vi "Sub Super Duper_2014 05 29_JWa.vi"(0 "VISA resource name":refnum<visa-resource-name>="GPIB0::17::INSTR", 1 "Sample Properties:":T9 {"Date Created" format="%<%Y/%m/%d>T"}, 2 "Gated SMU4 is...":bool, 3 "TRF Cluster":T10={"Step 4"=-38.0, "# of Loops"=1.0, "Transfer 2"=FALSE, "Start 4"=-2.0, "Total Points 2"=2, "Start 3"=40.0, "Stop 2"=-40.0, "Step 3"=-1.0, "Loop Step"=0.0, "Integration Time 3"=0, "Loop Wait"=0.0, "First Step"=0.0} {"Loop Wait" format="%<%H:%M:%S>t"; "Integration Time 3" scale=0.0..2.0; "Step 3" format="%.2f"; "Stop 2" format="%.2f"; "Start 3" format="%.2f"; "Start 4" format="%.2f"; "Step 4" format="%.2f"}, 4 "TSP Cluster":T11={"Transport"=FALSE, "Start 2"=0.0, "Stop 3"=-60.0, "Step 2"=-1.0, "Start"=0.0, "Step"=-10.0, "Total Points"=7, "Integration Time"=0} {"Integration Time" scale=0.0..2.0; "Step" format="%.2f"; "Start" format="%.2f"; "Step 2" format="%.2f"; "Stop 3" format="%.2f"; "Start 2" format="%.2f"}, 5 "Compliance Cluster":T6={"Var1 sweep settings"={"sweep spacing (linear: 0)"=0, "sweep mode"=FALSE, "compliance (V)"=100.0, "compliance (A)"=0.001}, "Var1 sweep settings 2"={"sweep spacing (linear: 0)"=0, "sweep mode"=FALSE, "compliance (V)"=100.0, "compliance (A)"=0.001}, "Var2 step settings 2"={"compliance (A)"=0.001, "compliance (V)"=100.0}, "Var2 step settings"={"compliance (A)"=0.001, "compliance (V)"=100.0}} {"Var2 step settings"."compliance (V)" format="%.2f"; "Var2 step settings"."compliance (A)" format="%^.2e"; "Var2 step settings 2"."compliance (V)" format="%.2f"; "Var2 step settings 2"."compliance (A)" format="%^.2e"; "Var1 sweep settings 2"."compliance (A)" format="%^.2e"; "Var1 sweep settings 2"."compliance (V)" format="%.2f"; "Var1 sweep settings 2"."sweep spacing (linear: 0)" items=["linear", "log 10", "log 25", "log 50"]; "Var1 sweep settings"."compliance (A)" format="%^.2e"; "Var1 sweep settings"."compliance (V)" format="%.2f"; "Var1 sweep settings"."sweep spacing (linear: 0)" items=["linear", "log 10", "log 25", "log 50"]}, 6 "Light Bathe Cluster":T2={"TG to BG:  "=FALSE, "TG to BG Durration"=120.0, "TRF to TSP:   "=FALSE, "TRF to TSP Duration"=120.0, "Post Measure: "=FALSE, "TG to BG (TSP):"=FALSE, "TG to BG Durration 3"=120.0} {"TG to BG Durration 3" format="%<%H:%M:%S>t"; "TRF to TSP Duration" format="%<%H:%M:%S>t"; "TG to BG Durration" format="%<%H:%M:%S>t"}, 7 "error in":errorcluster, 8 "Saved Folder:":path=path "C:/1DATA/2011", 9 "Wait Cluster":T5 {"Wait Time (s)" format="%.1g"; "Wait Countdown" format="%<%H:%M:%S%1u>t"}, 11 "TG Dielectric Prop":T1, 13 "Stop \nCountdown":bool, 15 "Loop Count":dbl, 16 "Gate Current Cluster":T3={"Gate Current (TSP)"={"Y2 axis on/off"=FALSE, "MINIMUM"=0.0, "MAXIMUM"=1.0, "Variable name"="Ig", "LIN or LOG axis"="LIN"}, "Gate Current (TRF)"={"Y2 axis on/off"=FALSE, "MINIMUM"=0.0, "MAXIMUM"=1.0, "Variable name"="Ig", "LIN or LOG axis"="LIN"}} {"Gate Current (TSP)"."MAXIMUM" format="%.9f"; "Gate Current (TSP)"."MINIMUM" format="%.9f"; "Gate Current (TRF)"."MAXIMUM" format="%.9f"; "Gate Current (TRF)"."MINIMUM" format="%.9f"}, 17 "Dielectric Constant (BG)":dbl) -> (12 "Status Indicator":bool, 14 "Vt Cluster":T4 {"Id Max" format="%.3g"; "Vt Max" format="%.3g"; "Vt Min" format="%.3g"; "Vt Ratio" format="%.3g"}, 20 "VISA resource name out":refnum<visa-resource-name>, 21 "TRF Path":path, 23 "TSP Path":path, 24 "Graph Cluster":T7, 25 "Char Cluster":T8 {"Mobility-Lin" format="%#_4e"; "On/Off" format="%#_4e"; "Mobility-Sat" format="%#_4e"}, 27 "error out":errorcluster)   [LabVIEW 2012]
uses:
  <vilib>/Platform/TimedLoop/XDataNode/wakeup.ctl
  <vilib>/Platform/TimedLoop/XDataNode/XDNodeRunTimeDep.lvlib
  <vilib>/Platform/TimedLoop/XDataNode/nitl_modes.ctl
  <vilib>/Platform/TimedLoop/XDataNode/timing_clust.ctl
  <vilib>/Platform/TimedLoop/XDataNode/XDataNode.xnode
panel:
  in  "Ambient Temp (Y/N)":bool=TRUE
  out "LKG Path":path
  # "Vg Sweep"
  # "Vd Step"
  # "Loops and Integration Time"
  # "Device Characteristics"
  # "Light Bath is..."
  # "Duration (hh:mm:ss)"
  # "Sample Properties:"
  # "%"
  # "nm"
  # "Device Properties:"
  # "um"
  # "um"
  # "Vg Step"
  # "Vd Step"
  # "Integration Time"
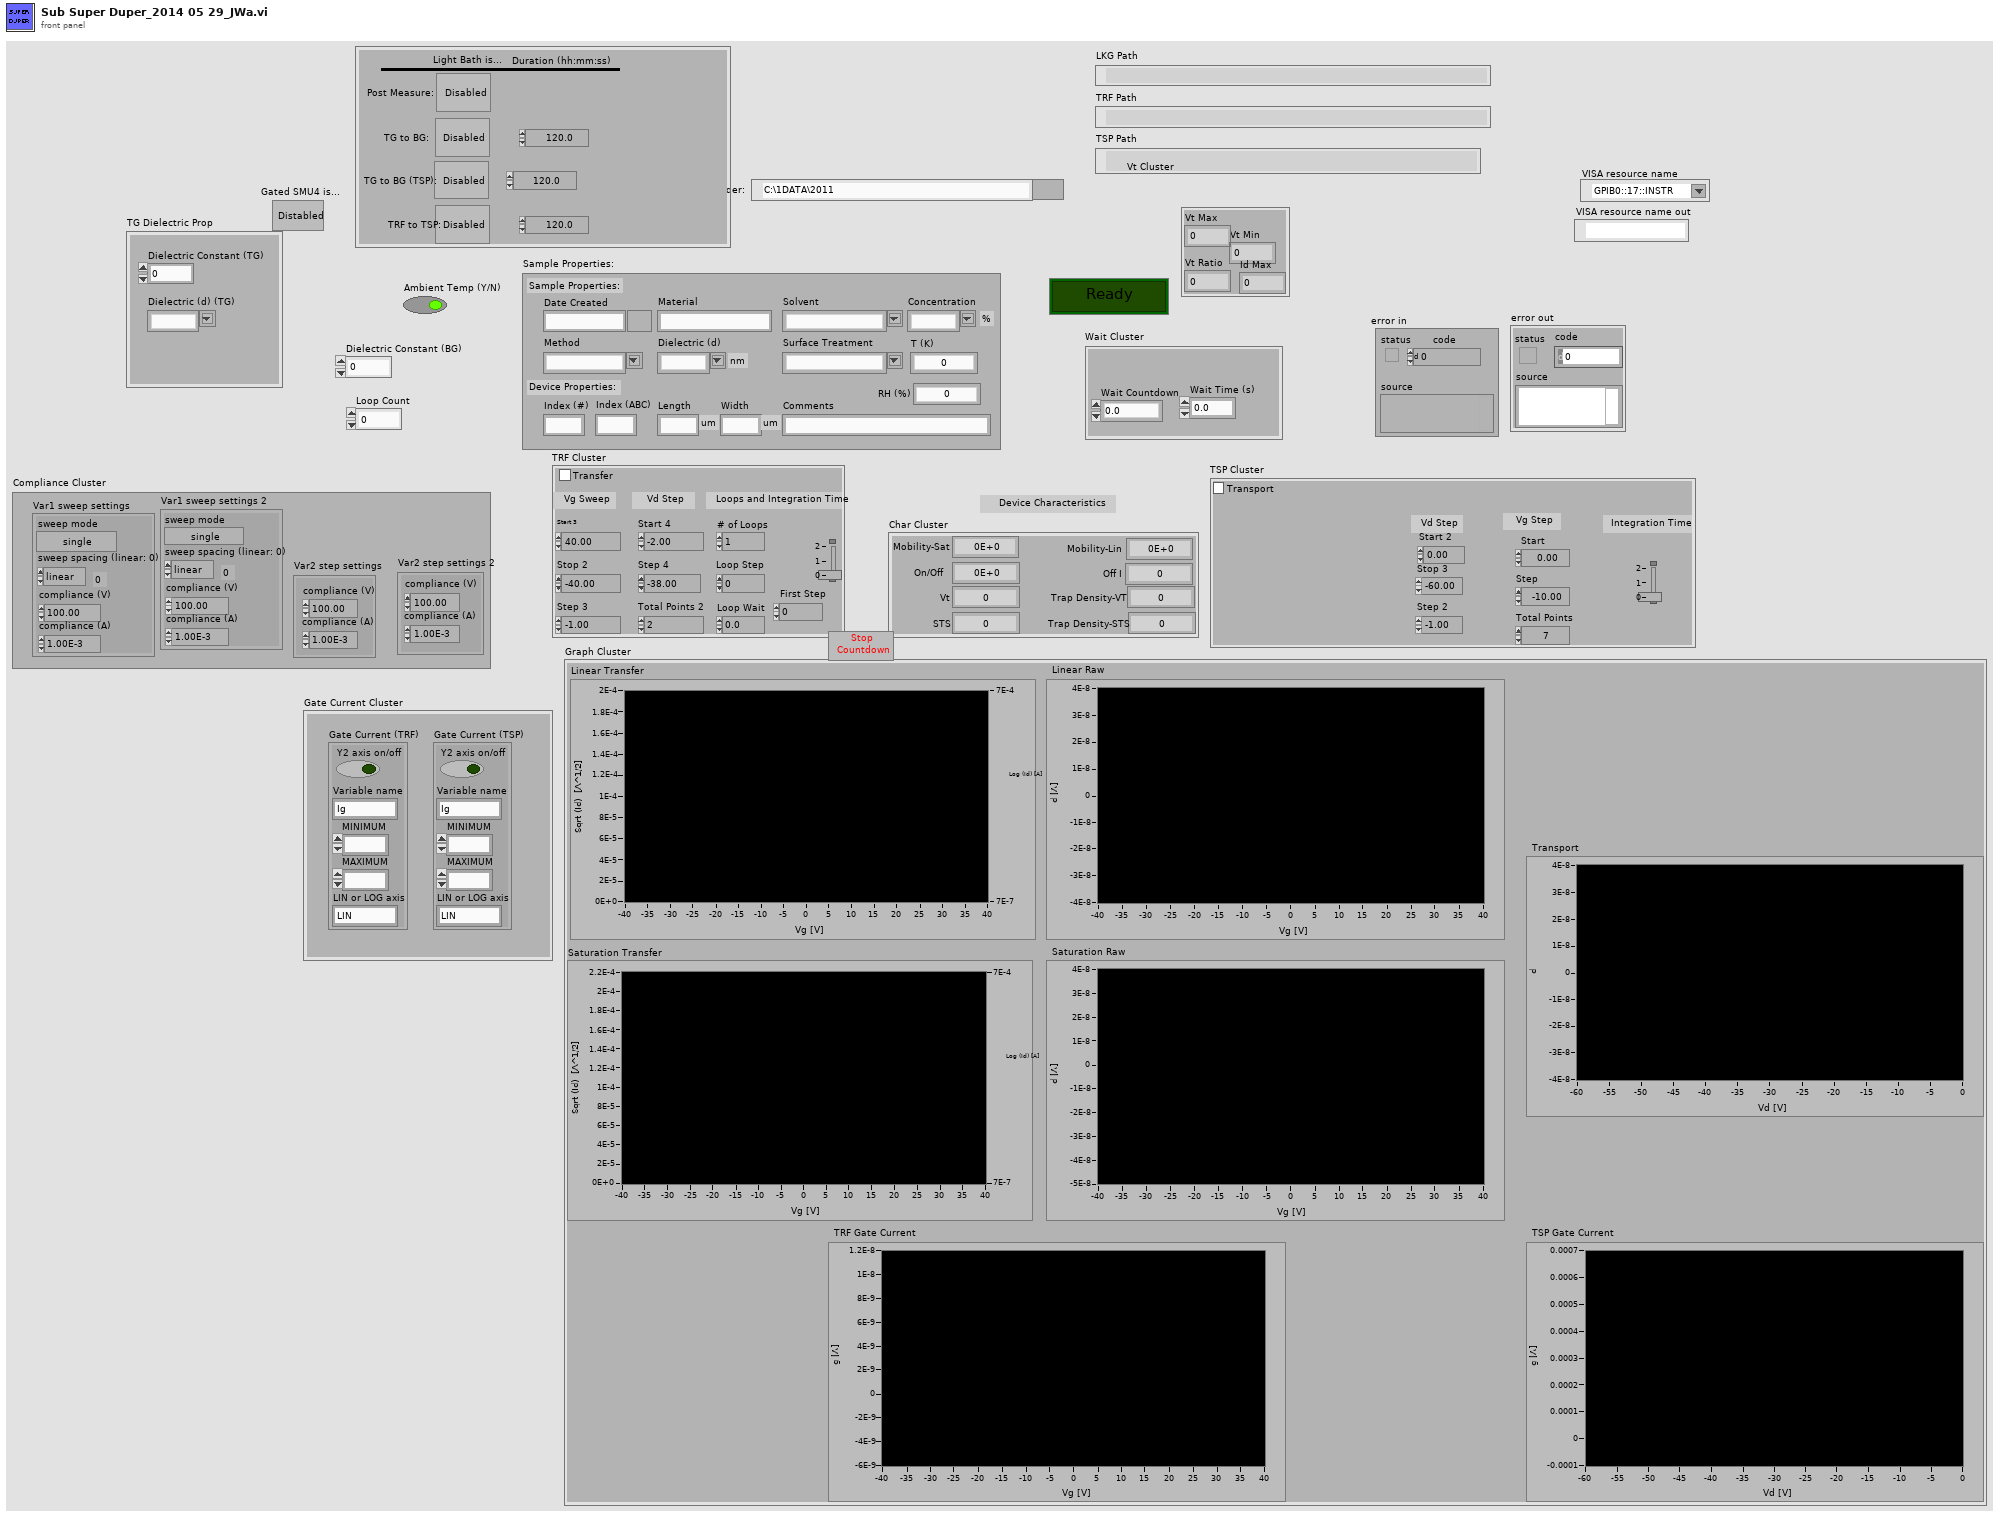
[diagram p1: front panel]
types:
  T1 = cluster{"Dielectric Constant (TG)":dbl, "Dielectric (d) (TG)":string}
  T2 = cluster{"TG to BG:  ":bool, "TG to BG Durration":dbl, "TRF to TSP:   ":bool, "TRF to TSP Duration":dbl, "Post Measure: ":bool, "TG to BG (TSP):":bool, "TG to BG Durration 3":dbl}
  T3 = cluster{"Gate Current (TSP)":cluster{"Y2 axis on/off":bool, "MINIMUM":ext, "MAXIMUM":ext, "Variable name":string, "LIN or LOG axis":string}, "Gate Current (TRF)":cluster{"Y2 axis on/off":bool, "MINIMUM":ext, "MAXIMUM":ext, "Variable name":string, "LIN or LOG axis":string}}
  T4 = cluster{"Vt Max":i32, "Vt Min":i32, "Vt Ratio":i32, "Id Max":i32}
  T5 = cluster{"Wait Countdown":dbl, "Wait Time (s)":dbl}
  T6 = cluster{"Var1 sweep settings":cluster{"sweep spacing (linear: 0)":u16, "sweep mode":bool, "compliance (V)":dbl, "compliance (A)":dbl}, "Var1 sweep settings 2":cluster{"sweep spacing (linear: 0)":u16, "sweep mode":bool, "compliance (V)":dbl, "compliance (A)":dbl}, "Var2 step settings 2":cluster{"compliance (A)":dbl, "compliance (V)":dbl}, "Var2 step settings":cluster{"compliance (A)":dbl, "compliance (V)":dbl}}
  T7 = cluster{"Linear Transfer":cluster{dbl[], "trace":dbl[]}[], "Linear Raw":cluster{dbl[], dbl[]}[], "Saturation Transfer":cluster{dbl[], "trace":dbl[]}[], "Saturation Raw":cluster{dbl[], dbl[]}[], "Transport":cluster{dbl[], dbl[]}[], "TRF Gate Current":cluster{dbl[], dbl[]}[], "TSP Gate Current":cluster{dbl[], dbl[]}[]}
  T8 = cluster{"Mobility-Sat":dbl, "Mobility-Lin":dbl, "On/Off ":dbl, "Off I":dbl, "Vt":dbl, "STS":dbl, "Trap Density-VT":dbl, "Trap Density-STS":dbl}
  T9 = cluster{"Date Created":timestamp, "Material":string, "Solvent":string, "Concentration":string, "Method":string, "Dielectric (d)":string, "Index (#)":string, "Index (ABC)":string, "Length":string, "Width":string, "Surface Treatment":string, "Comments":string, "T (K)":dbl, "RH (%)":dbl}
  T10 = cluster{"Step 4":dbl, "# of Loops":dbl, "Transfer 2":bool, "Start 4":dbl, "Total Points 2":u16, "Start 3":dbl, "Stop 2":dbl, "Step 3":dbl, "Loop Step":dbl, "Integration Time 3":u32, "Loop Wait":dbl, "First Step":dbl}
  T11 = cluster{"Transport":bool, "Start 2":dbl, "Stop 3":dbl, "Step 2":dbl, "Start":dbl, "Step":dbl, "Total Points":u16, "Integration Time":u32}
  T12 = typedef "XDNodeRunTimeDep.lvlib/timing_clust.ctl" = cluster{"Expected End [f-1]":u64, "Actual End [f-1]":u64, "Finished Late? [f-1]":bool, "Expected End [i-1]":u64, "Actual End [i-1]":u64, "Finished Late? [i-1]":bool, "Expected Start [i]":u64, "Actual Start [i]":u64, "Expected Start [f]":u64, "Actual Start [f]":u64, "Source Name":string, "Structure Name":string, "Period":i64, "Deadline":i64, "Offset":i64, "Start":i64, "Priority":i32, "Timeout":i32, "Mode":T13, "Wakeup Reason":T14, "Error":errorcluster, "Source Type":string, "Secondary Source Type":string, "Global End Time":u64, "Global Start Time":u64, "Frame Duration":u64, "Iteration Duration":u64, "Assigned CPU":i32, "I/O Scan Engine Mode":u32}
  T13 = typedef "XDNodeRunTimeDep.lvlib/nitl_modes.ctl" = enum32{"No Change", "Process missed periods, maintain original phase", "Discard missed periods, maintain original phase", "Process missed periods, ignore original phase", "Discard missed periods, ignore original phase"}
  T14 = typedef "XDNodeRunTimeDep.lvlib/wakeup.ctl" = enum32{"Normal", "Aborted", "Asynchronous wakeup", "Timing source error", "Timed loop error", "Timeout"}
  T15 = cluster{"sweep spacing (linear: 0)":u16, "sweep mode":bool, "compliance (V)":dbl, "compliance (A)":dbl}
  T16 = cluster{"compliance (A)":dbl, "compliance (V)":dbl}
  T17 = cluster{"Y2 axis on/off":bool, "MINIMUM":ext, "MAXIMUM":ext, "Variable name":string, "LIN or LOG axis":string}
  T18 = cluster{"Start 3":dbl, "Stop 2":dbl, "Step 3":dbl, "sweep spacing (linear: 0)":u16, "sweep mode":bool, "compliance (V)":dbl, "compliance (A)":dbl}
  T19 = cluster{"compliance (A)":dbl, "compliance (V)":dbl, "Start 4":dbl, "Total Points 2":u16, dbl}
  T20 = cluster{"Vt Max":i32, "Vt Min":i32, "Vt Ratio":i32, "Id Max":dbl}
  T21 = cluster{"Mobility-Sat":dbl, "Mobility-Lin":dbl, "On/Off Current":dbl, "Off I":dbl, "Vt":dbl, "STS":dbl, "Trap Density-VT":dbl, "Trap Density-STS":dbl}
  T22 = cluster{"Linear Sqrt":cluster{dbl[], "trace":dbl[]}[], "Linear Log":cluster{dbl[], "trace":dbl[]}[], "Linear Raw":cluster{dbl[], dbl[]}[], "Saturation Sqrt":cluster{dbl[], "trace":dbl[]}[], "Saturation Log":cluster{dbl[], "trace":dbl[]}[], "Saturation Raw":cluster{dbl[], "trace":dbl[]}[], "Gate Current":cluster{dbl[], "trace":dbl[]}[]}
  T23 = cluster{"Start 2":dbl, "Stop 3":dbl, "Step 2":dbl, "sweep spacing (linear: 0)":u16, "sweep mode":bool, "compliance (V)":dbl, "compliance (A)":dbl}
  T24 = cluster{"compliance (A)":dbl, "compliance (V)":dbl, "Start":dbl, "Total Points":u16, "Step":dbl}
  T25 = cluster{"Transport":cluster{dbl[], dbl[]}[], "Gate Current":cluster{dbl[], dbl[]}[]}
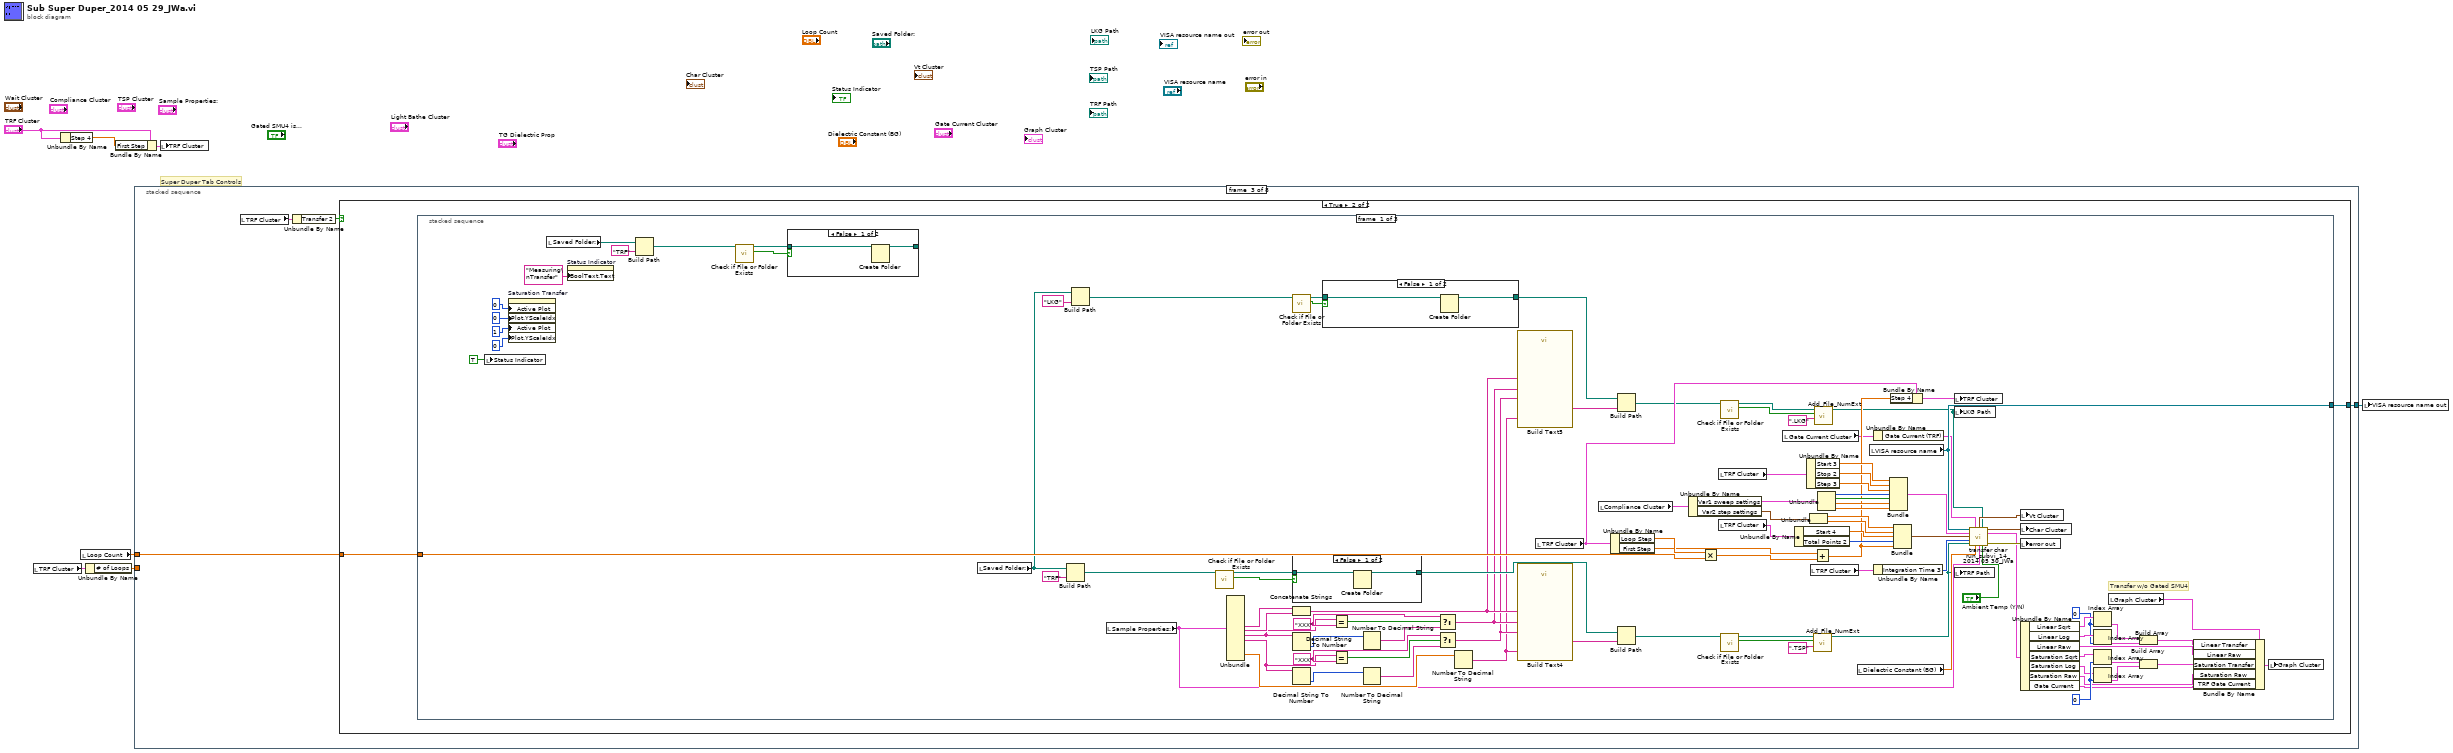
[diagram p0: block diagram]
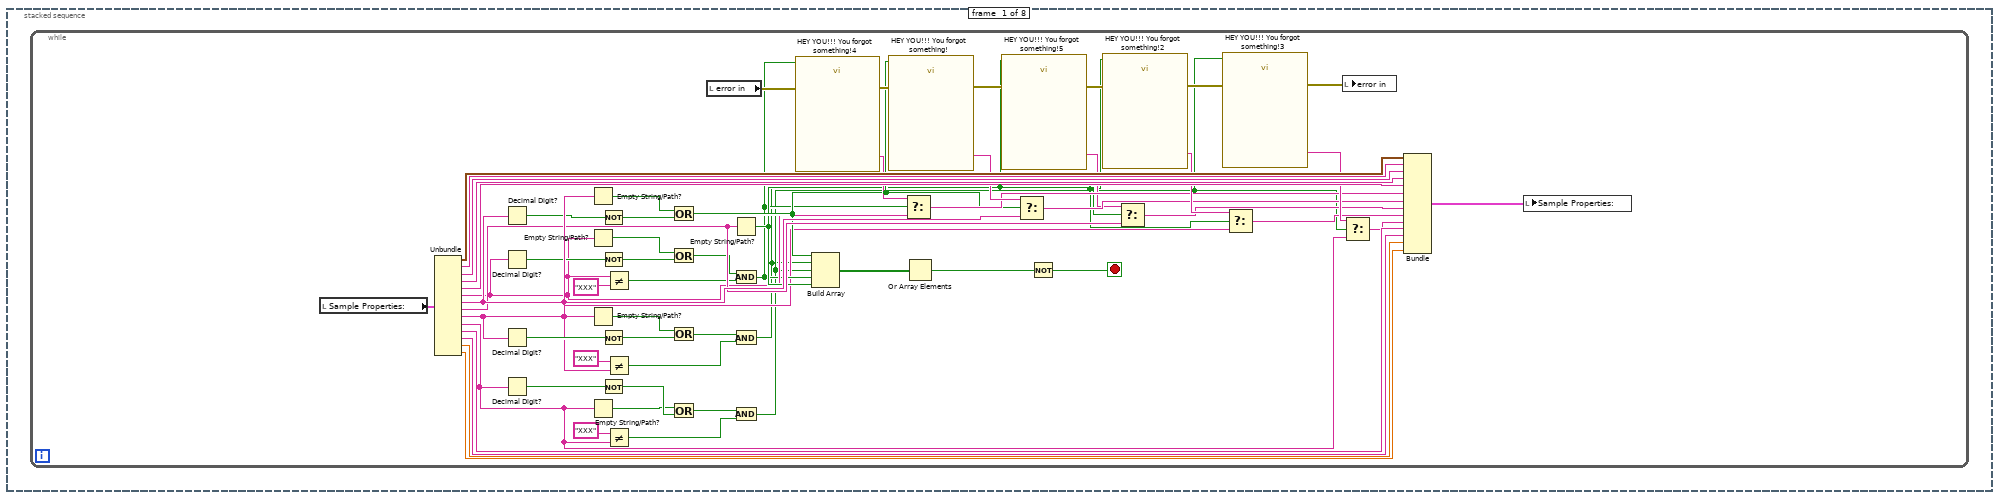
[diagram p2: hidden frame]
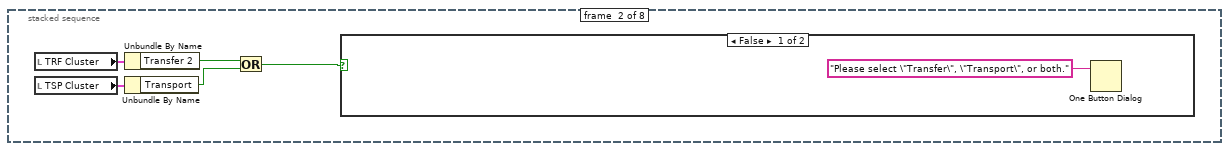
[diagram p3: hidden frame]
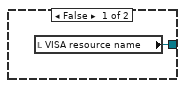
[diagram p5: hidden frame]
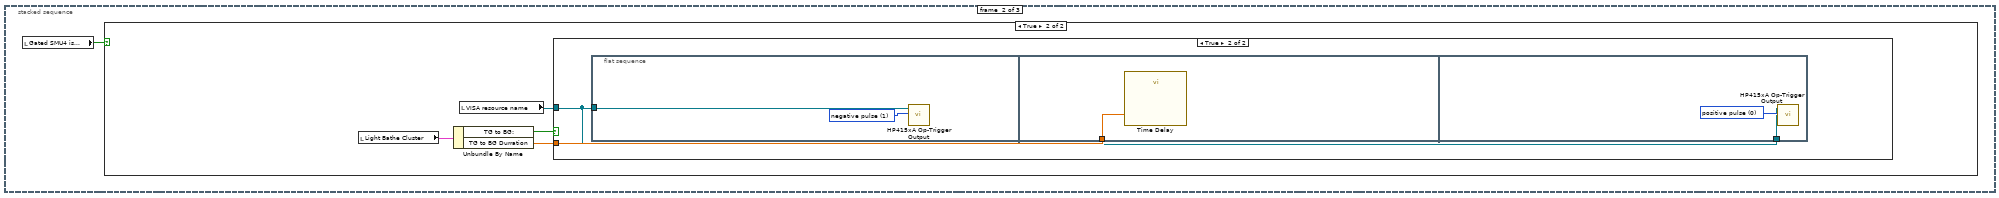
[diagram p9: hidden frame]
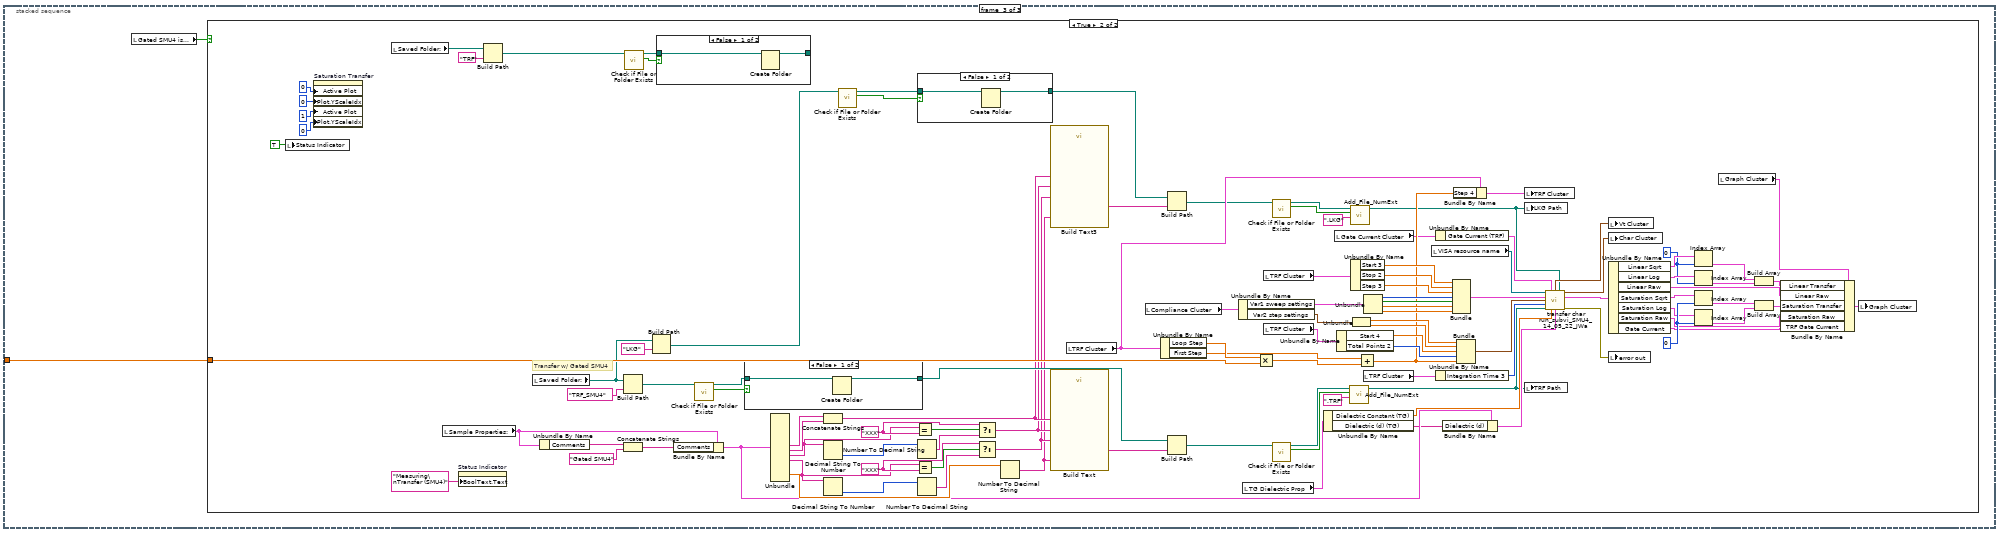
[diagram p12: hidden frame]
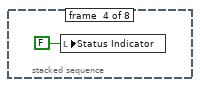
[diagram p17: hidden frame]
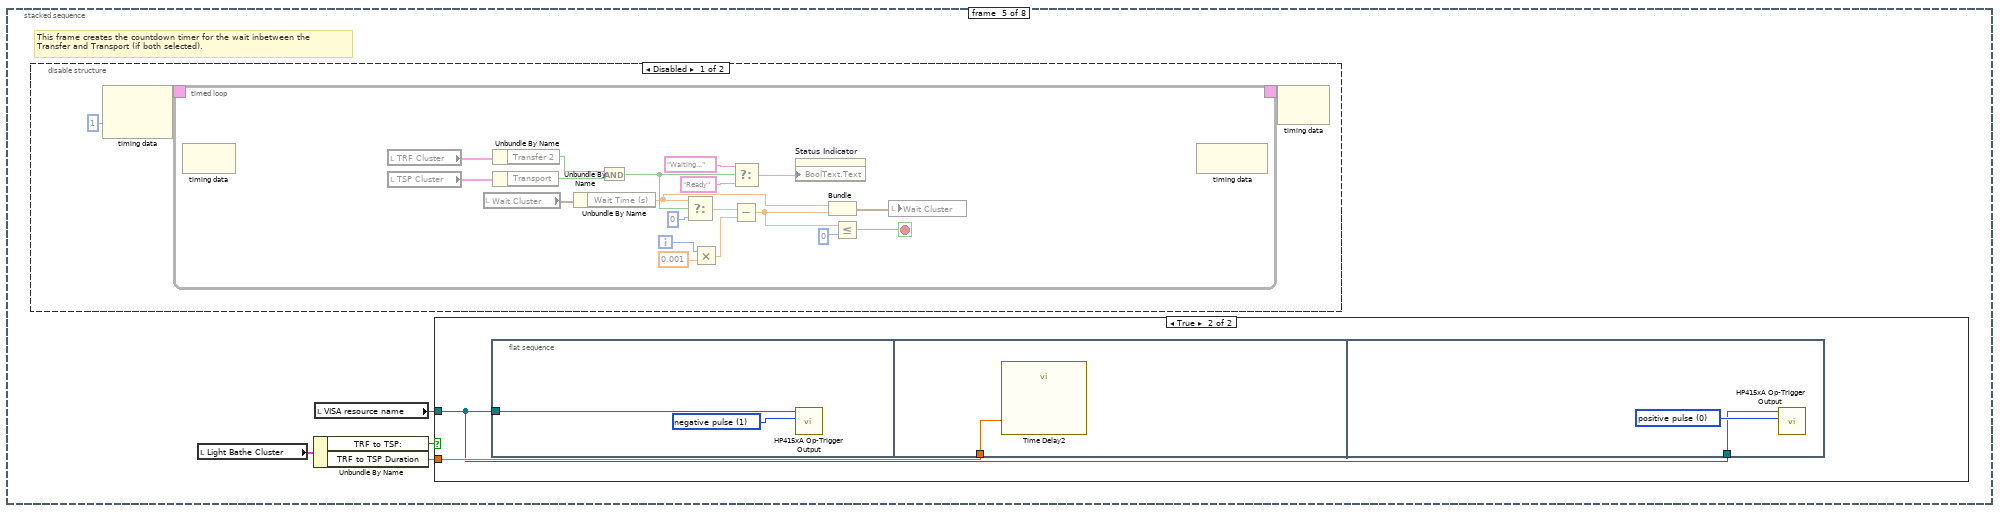
[diagram p18: hidden frame]
diagram:
  # "Super Duper Tab Controls"
  n1 = local read "TRF Cluster"() -> (w4:T10)
  n2 = Unbundle By Name("TRF Cluster") -> ("Step 4"=w5:dbl)
  n3 = local read "Loop Count"() -> (w1:dbl)
  n4 = Unbundle By Name(w4) -> ("# of Loops"=w3:dbl)
  n5 = Bundle By Name(cluster="TRF Cluster", "First Step"=w5) -> (w7:T10)
  n6 = stacked-sequence {
    tunnel: w1 -> [_ _ w78 _ _ _ _ w516]
    tunnel: w3 -> [_ _ _ _ _ _ _ w515]
    tunnel: [_ _ w75 _ _ _ _ _] -> w2
    frame #0 {
      n7 = while {
        stop <- w34 stop-if-true
        n8 = local read "Sample Properties:"() -> (w63:T9)
        n9 = Unbundle(w63) -> ("Date Created"=w64:timestamp, "Material"=w65:string, "Solvent"=w66:string, "Concentration"=w67:string, "Method"=w68:string, "Dielectric (d)"=w23:string, "Index (#)"=w53:string, "Index (ABC)"=w50:string, "Length"=w18:string, "Width"=w11:string, "Surface Treatment"=w56:string, "Comments"=w48:string, "T (K)"=w9:dbl, "RH (%)"=w8:dbl)
        n10 = Decimal Digit?(1:w53) -> (0:w44:bool)
        n11 = Decimal Digit?(1:w23) -> (0:w31:bool)
        n12 = Decimal Digit?(1:w18) -> (0:w33:bool)
        n13 = Decimal Digit?(1:w11) -> (0:w32:bool)
        n14 = Empty String/Path?(string/path=w53) -> (empty?=w52:bool)
        n15 = Empty String/Path?(string/path=w23) -> (empty?=w25:bool)
        n16 = Empty String/Path?(string/path=w18) -> (empty?=w27:bool)
        n17 = Empty String/Path?(string/path=w11) -> (empty?=w26:bool)
        n18 = Not(x=w44) -> (.not. x?=w43:bool)
        n19 = Not(x=w31) -> (.not. x?=w28:bool)
        n20 = Not(x=w33) -> (.not. x?=w30:bool)
        n21 = Not(x=w32) -> (.not. x?=w29:bool)
        n22 = Not Equal?(x=w23, y="XXX") -> (x != y?=w22:bool)
        n23 = Not Equal?(x="XXX", y=w18) -> (x != y?=w17:bool)
        n24 = Not Equal?(x="XXX", y=w11) -> (x != y?=w15:bool)
        n25 = Or(x=w52, y=w43) -> (x .or. y?=w38:bool)
        n26 = Or(x=w25, y=w28) -> (x .or. y?=w21:bool)
        n27 = Or(x=w27, y=w30) -> (x .or. y?=w16:bool)
        n28 = Or(x=w26, y=w29) -> (x .or. y?=w14:bool)
        n29 = local read "error in"() -> (w40:errorcluster)
        n30 = Empty String/Path?(string/path=w50) -> (empty?=w37:bool)
        n31 = And(x=w21, y=w22) -> (x .and. y?=w20:bool)
        n32 = And(x=w16, y=w17) -> (x .and. y?=w10:bool)
        n33 = And(x=w14, y=w15) -> (x .and. y?=w13:bool)
        n34 = call "HEY YOU!!! You forgot something!4"("Enable"=w20, "error in (no error)"=w40) -> ("Dielectric (d)"=w55:string, "error out"=w39:errorcluster)  [unwired: 15 in, 1 out]
        n35 = Build Array(w38, w10, w13, w20, w37) -> (w36:bool[])
        n36 = call "HEY YOU!!! You forgot something!"("Enable"=w38, "error in (no error)"=w39) -> ("Index (#)"=w62:string, "error out"=w42:errorcluster)  [unwired: 15 in, 1 out]
        n37 = Select(t=w55, s=w20, f=w23) -> (s? t:f=w54:string)
        n38 = Or Array Elements(Boolean array=w36) -> (logical OR=w35:bool)
        n39 = call "HEY YOU!!! You forgot something!5"("Enable"=w37, "error in (no error)"=w42) -> ("Index (ABC)"=w51:string, "error out"=w41:errorcluster)  [unwired: 15 in, 1 out]
        n40 = Select(t=w62, s=w38, f=w53) -> (s? t:f=w59:string)
        n41 = Not(x=w35) -> (.not. x?=w34:bool)
        n42 = call "HEY YOU!!! You forgot something!2"("Enable"=w10, "error in (no error)"=w41) -> ("Length"=w61:string, "error out"=w58:errorcluster)  [unwired: 15 in, 1 out]
        n43 = Select(t=w51, s=w37, f=w50) -> (s? t:f=w49:string)
        n44 = call "HEY YOU!!! You forgot something!3"("Enable"=w13, "error in (no error)"=w58) -> ("Width"=w60:string, "error out"=w57:errorcluster)  [unwired: 15 in, 1 out]
        n45 = Select(t=w61, s=w10, f=w18) -> (s? t:f=w47:string)
        n46 = local write "error in"(w57) -> ()
        n47 = Select(t=w60, s=w13, f=w11) -> (s? t:f=w46:string)
        n48 = Bundle("Date Created"=w64, "Material"=w65, "Solvent"=w66, "Concentration"=w67, "Method"=w68, "Dielectric (d)"=w54, "Index (#)"=w59, "Index (ABC)"=w49, "Length"=w47, "Width"=w46, "Surface Treatment"=w56, "Comments"=w48, "T (K)"=w9, "RH (%)"=w8) -> (w45:T9)  [unwired: 1 in]
        n49 = local write "Sample Properties:"(w45) -> ()
      }
    }
    frame #1 {
      n50 = local read "TRF Cluster"() -> (w72:T10)
      n51 = local read "TSP Cluster"() -> (w70:T11)
      n52 = Unbundle By Name(w72) -> ("Transfer 2"=w71:bool)
      n53 = Unbundle By Name(w70) -> ("Transport"=w69:bool)
      n54 = Or(x=w71, y=w69) -> (x .or. y?=w73:bool)
      n55 = case shown="False" w73 {
        frame False {
          n56 = One Button Dialog(message="Please select \"Transfer\", \"Transport\", or both.") -> ()  [unwired: 1 in, 1 out]
        }
        frame True {
        }
      }
    }
    frame #2 {
      n57 = local read "TRF Cluster"() -> (w76:T10)
      n58 = Unbundle By Name(w76) -> ("Transfer 2"=w77:bool)
      n59 = case shown="True" w77 {
        tunnel: w78 -> [_ w81]
        tunnel: [w79 w80] -> w75
        frame False {
          n60 = local read "VISA resource name"() -> (w79:refnum<visa-resource-name>)
        }
        frame True {
          n61 = stacked-sequence {
            tunnel: w81 -> [w186 _ w209]
            tunnel: [w185 _ _] -> w80
            frame #0 {
              w119 = 0
              w125 = 0
              w166 = "XXX"
              w169 = "XXX"
              # "Transfer w/o Gated SMU4"
              n62 = local write "Status Indicator"(TRUE) -> ()
              n63 = property on="Saturation Transfer" class="XYGraph (strict)"("Active Plot"=0, "Plot.YScaleIdx"=0, "Active Plot"=1, "Plot.YScaleIdx"=0) -> ()  [unwired: 2 in, 2 out]
              n64 = local read "Saved Folder:"() -> (w112:path)
              n65 = property on="Status Indicator" class="Bool (strict)"("BoolText.Text"="Measuring\nTransfer") -> ()  [unwired: 2 in, 2 out]
              n66 = Build Path(base path=w112, name or relative path="TRF") -> (appended path=w110:path)
              n67 = call <vilib>:"Check if File or Folder Exists.vi"("path"=w110) -> ("file or folder exists?"=w108:bool, "dup path"=w109:path)  [unwired: 8 in, 1 out]
              n68 = case shown="False" w108 {
                tunnel: w109 -> [w191 w192]
                tunnel: [w190 w192] -> _
                frame False {
                  n69 = Create Folder(path (use dialog)=w191) -> (created path=w190:path)  [unwired: 2 in, 2 out]
                }
                frame True {
                }
              }
              n70 = local read "Saved Folder:"() -> (w106:path)
              n71 = Build Path(base path=w106, name or relative path="TRF") -> (appended path=w159:path)
              n72 = Build Path(base path=w106, name or relative path="LKG") -> (appended path=w102:path)
              n73 = local read "Sample Properties:"() -> (w91:T9)
              n74 = call <vilib>:"Check if File or Folder Exists.vi"("path"=w159) -> ("file or folder exists?"=w161:bool, "dup path"=w160:path)  [unwired: 8 in, 1 out]
              n75 = Unbundle(w91) -> ("Index (#)"=w175:string, "Index (ABC)"=w174:string, "Length"=w163:string, "Width"=w165:string, "T (K)"=w142:dbl)  [unwired: 9 out]
              n76 = call <vilib>:"Check if File or Folder Exists.vi"("path"=w102) -> ("file or folder exists?"=w103:bool, "dup path"=w104:path)  [unwired: 8 in, 1 out]
              n77 = case shown="False" w161 {
                tunnel: w160 -> [w194 w195]
                tunnel: [w193 w195] -> w158
                frame False {
                  n78 = Create Folder(path (use dialog)=w194) -> (created path=w193:path)  [unwired: 2 in, 2 out]
                }
                frame True {
                }
              }
              n79 = Concatenate Strings(w175, w174) -> (w99:string)
              n80 = Decimal String To Number(string=w163) -> (number=w172:i32)  [unwired: 2 in, 1 out]
              n81 = Decimal String To Number(string=w165) -> (number=w171:i32)  [unwired: 2 in, 1 out]
              n82 = case shown="False" w103 {
                tunnel: w104 -> [w188 w189]
                tunnel: [w187 w189] -> w95
                frame False {
                  n83 = Create Folder(path (use dialog)=w188) -> (created path=w187:path)  [unwired: 2 in, 2 out]
                }
                frame True {
                }
              }
              n84 = Equal?(x=w163, y=w169) -> (x = y?=w170:bool)
              n85 = Equal?(x=w165, y=w166) -> (x = y?=w167:bool)
              n86 = Number To Decimal String(number=w172) -> (decimal integer string=w168:string)  [unwired: 1 in]
              n87 = Number To Decimal String(number=w171) -> (decimal integer string=w164:string)  [unwired: 1 in]
              n88 = Select(t=w169, s=w170, f=w168) -> (s? t:f=w98:string)
              n89 = Select(t=w166, s=w167, f=w164) -> (s? t:f=w97:string)
              n90 = Number To Decimal String(number=w142) -> (decimal integer string=w96:string)  [unwired: 1 in]
              n91 = call "Build Text5"("T"=w96, "Index"=w99, "Length"=w98, "Width"=w97) -> ("Result"=w100:string)  [unwired: 10 in, 1 out]
              n92 = call "Build Text4"("T"=w96, "Index"=w99, "Length"=w98, "Width"=w97) -> ("Result"=w178:string)  [unwired: 10 in, 1 out]
              n93 = local read "TRF Cluster"() -> (w136:T10)
              n94 = local read "Compliance Cluster"() -> (w145:T6)
              n95 = Unbundle By Name(w136) -> ("Loop Step"=w139:dbl, "First Step"=w138:dbl)
              n96 = Build Path(base path=w95, name or relative path=w100) -> (appended path=w101:path)
              n97 = Build Path(base path=w158, name or relative path=w178) -> (appended path=w173:path)
              n98 = Unbundle By Name(w145) -> ("Var1 sweep settings"=w143:T15, "Var2 step settings"=w144:T16)
              n99 = Multiply(x=w139, y=w186) -> (x*y=w141:dbl)
              n100 = local read "TRF Cluster"() -> (w150:T10)
              n101 = local read "TRF Cluster"() -> (w153:T10)
              n102 = call <vilib>:"Check if File or Folder Exists.vi"("path"=w101) -> ("file or folder exists?"=w83:bool, "dup path"=w84:path)  [unwired: 8 in, 1 out]
              n103 = call <vilib>:"Check if File or Folder Exists.vi"("path"=w173) -> ("file or folder exists?"=w88:bool, "dup path"=w87:path)  [unwired: 8 in, 1 out]
              n104 = local read "Gate Current Cluster"() -> (w94:T3)
              n105 = Unbundle By Name(w153) -> ("Start 4"=w152:dbl, "Total Points 2"=w151:u16)
              n106 = Unbundle By Name(w150) -> ("Start 3"=w149:dbl, "Stop 2"=w148:dbl, "Step 3"=w147:dbl)
              n107 = Unbundle(w144) -> ("compliance (A)"=w180:dbl, "compliance (V)"=w179:dbl)
              n108 = local read "TRF Cluster"() -> (w146:T10)
              n109 = Add(x=w138, y=w141) -> (x+y=w137:dbl)
              n110 = call "Add_File_NumExt.vi"("Extension"=".TSP" ("string"), "file or folder exists?"=w88, "Path In"=w87) -> ("Path Out"=w90:path)  [unwired: 8 in]
              n111 = call "Add_File_NumExt.vi"("Extension"=".LKG" ("string"), "file or folder exists?"=w83, "Path In"=w84) -> ("Path Out"=w86:path)  [unwired: 8 in]
              n112 = Unbundle(w143) -> ("sweep spacing (linear: 0)"=w184:u16, "sweep mode"=w183:bool, "compliance (V)"=w182:dbl, "compliance (A)"=w181:dbl)
              n113 = local read "Dielectric Constant (BG)"() -> (w92:dbl)
              n114 = local read "VISA resource name"() -> (w185:refnum<visa-resource-name>)
              n115 = Unbundle By Name(w94) -> ("Gate Current (TRF)"=w93:T17)
              n116 = Unbundle By Name(w146) -> ("Integration Time 3"=w133:u32)
              n117 = Bundle("Start 3"=w149, "Stop 2"=w148, "Step 3"=w147, "sweep spacing (linear: 0)"=w184, "sweep mode"=w183, "compliance (V)"=w182, "compliance (A)"=w181) -> (w135:T18)  [unwired: 1 in]
              n118 = Bundle By Name(cluster=w136, "Step 4"=w137) -> (w140:T10)
              n119 = Bundle("compliance (A)"=w180, "compliance (V)"=w179, "Start 4"=w152, "Total Points 2"=w151, w137) -> (w134:T19)  [unwired: 1 in]
              n120 = local write "TRF Cluster"(w140) -> ()
              n121 = local write "LKG Path"(w86) -> ()
              n122 = local write "TRF Path"(w90) -> ()
              n123 = call "transfer char run_subvi_14_2014 05 30_JWa.vi"("VISA session"=w185, "Y2 axis settings"=w93, "LKG Path"=w86, "Var1 sweep settings"=w135, "Var2 step settings"=w134, "integration time"=w133, "Input Path"=w90, "Dielectric Constant"=w92, "Sample Properties:"=w91, "Ambient Temp (Y/N)"="Ambient Temp (Y/N)") -> ("Check Cluster"=w130:T20, "Output"=w131:T21, "Graph Cluster"=w129:T22, "Error In"=w132:errorcluster)  [unwired: 2 in]
              n124 = local write "Vt Cluster"(w130) -> ()
              n125 = local write "Char Cluster"(w131) -> ()
              n126 = local write "error out"(w132) -> ()
              n127 = Unbundle By Name(w129) -> ("Linear Sqrt"=w127:cluster{dbl[], "trace":dbl[]}[], "Linear Log"=w126:cluster{dbl[], "trace":dbl[]}[], "Linear Raw"=w115:cluster{dbl[], dbl[]}[], "Saturation Sqrt"=w118:cluster{dbl[], "trace":dbl[]}[], "Saturation Log"=w117:cluster{dbl[], "trace":dbl[]}[], "Saturation Raw"=w114:cluster{dbl[], "trace":dbl[]}[], "Gate Current"=w107:cluster{dbl[], "trace":dbl[]}[])
              n128 = Index Array(array=w127, index=w125) -> (element=w124:cluster{dbl[], "trace":dbl[]})
              n129 = Index Array(array=w126, index=w125) -> (element=w123:cluster{dbl[], "trace":dbl[]})
              n130 = Index Array(array=w118, index=w119) -> (element=w120:cluster{dbl[], "trace":dbl[]})
              n131 = Index Array(array=w117, index=w119) -> (element=w121:cluster{dbl[], "trace":dbl[]})
              n132 = local read "Graph Cluster"() -> (w128:T7)
              n133 = Build Array(w124, w123) -> (w122:cluster{dbl[], "trace":dbl[]}[])
              n134 = Build Array(w120, w121) -> (w116:cluster{dbl[], "trace":dbl[]}[])
              n135 = Bundle By Name(cluster=w128, "Linear Transfer"=w122, "Linear Raw"=w115, "Saturation Transfer"=w116, "Saturation Raw"=w114, "TRF Gate Current"=w107) -> (w113:T7)
              n136 = local write "Graph Cluster"(w113) -> ()
            }
            frame #1 {
              n137 = local read "Gated SMU4 is..."() -> (w196:bool)
              n138 = case shown="True" w196 {
                frame False {
                }
                frame True {
                  n139 = local read "Light Bathe Cluster"() -> (w200:T2)
                  n140 = Unbundle By Name(w200) -> ("TG to BG:"=w199:bool, "TG to BG Durration"=w198:dbl)
                  n141 = local read "VISA resource name"() -> (w197:refnum<visa-resource-name>)
                  n142 = case shown="True" w199 {
                    tunnel: w198 -> [_ w202]
                    tunnel: w197 -> [_ w201]
                    frame False {
                    }
                    frame True {
                      n143 = flat-sequence {
                        tunnel: w201 -> [w203]
                        tunnel: w202 -> [w205]
                        tunnel: w201 -> [w206]
                        frame #0 {
                          w204 = u32 1 items=["positive pulse  ", "negative pulse  ", "level high  ", "level low  "] ("trigger signal")
                          n144 = call "HP415xA Op-Trigger Output.vi"("trigger signal"=w204, "VISA session"=w203) -> ()  [unwired: 2 in, 1 out]
                        }
                        frame #1 {
                          n145 = call "Time Delay"("Delay Time (s)"=w205) -> ()  [unwired: 10 in, 1 out]
                        }
                        frame #2 {
                          w207 = u32 0 items=["positive pulse  ", "negative pulse  ", "level high  ", "level low  "] ("trigger signal")
                          n146 = call "HP415xA Op-Trigger Output.vi"("trigger signal"=w207, "VISA session"=w206) -> ()  [unwired: 2 in, 1 out]
                        }
                      }
                    }
                  }
                }
              }
            }
            frame #2 {
              n147 = local read "Gated SMU4 is..."() -> (w208:bool)
              n148 = case shown="True" w208 {
                tunnel: w209 -> [_ w276]
                frame False {
                }
                frame True {
                  w253 = 0
                  w259 = 0
                  w302 = "XXX"
                  w305 = "XXX"
                  # "Transfer w/ Gated SMU4"
                  n149 = local write "Status Indicator"(TRUE) -> ()
                  n150 = property on="Saturation Transfer" class="XYGraph (strict)"("Active Plot"=0, "Plot.YScaleIdx"=0, "Active Plot"=1, "Plot.YScaleIdx"=0) -> ()  [unwired: 2 in, 2 out]
                  n151 = local read "Saved Folder:"() -> (w246:path)
                  n152 = local read "Sample Properties:"() -> (w218:T9)
                  n153 = property on="Status Indicator" class="Bool (strict)"("BoolText.Text"="Measuring\nTransfer (SMU4)") -> ()  [unwired: 2 in, 2 out]
                  n154 = Build Path(base path=w246, name or relative path="TRF") -> (appended path=w244:path)
                  n155 = local read "Saved Folder:"() -> (w240:path)
                  n156 = Unbundle By Name(w218) -> ("Comments"=w226:string)
                  n157 = Build Path(base path=w240, name or relative path="TRF_SMU4") -> (appended path=w295:path)
                  n158 = Concatenate Strings(w226, "Gated SMU4" ("string")) -> (w224:string)
                  n159 = call <vilib>:"Check if File or Folder Exists.vi"("path"=w244) -> ("file or folder exists?"=w242:bool, "dup path"=w243:path)  [unwired: 8 in, 1 out]
                  n160 = Build Path(base path=w240, name or relative path="LKG") -> (appended path=w236:path)
                  n161 = case shown="False" w242 {
                    tunnel: w243 -> [w325 w326]
                    tunnel: [w324 w326] -> _
                    frame False {
                      n162 = Create Folder(path (use dialog)=w325) -> (created path=w324:path)  [unwired: 2 in, 2 out]
                    }
                    frame True {
                    }
                  }
                  n163 = Bundle By Name(cluster=w218, "Comments"=w224) -> (w221:T9)
                  n164 = call <vilib>:"Check if File or Folder Exists.vi"("path"=w295) -> ("file or folder exists?"=w297:bool, "dup path"=w296:path)  [unwired: 8 in, 1 out]
                  n165 = case shown="False" w297 {
                    tunnel: w296 -> [w328 w329]
                    tunnel: [w327 w329] -> w294
                    frame False {
                      n166 = Create Folder(path (use dialog)=w328) -> (created path=w327:path)  [unwired: 2 in, 2 out]
                    }
                    frame True {
                    }
                  }
                  n167 = Unbundle(w221) -> ("Index (#)"=w311:string, "Index (ABC)"=w310:string, "Length"=w299:string, "Width"=w301:string, "T (K)"=w278:dbl)  [unwired: 9 out]
                  n168 = Concatenate Strings(w311, w310) -> (w233:string)
                  n169 = Decimal String To Number(string=w299) -> (number=w308:i32)  [unwired: 2 in, 1 out]
                  n170 = Decimal String To Number(string=w301) -> (number=w307:i32)  [unwired: 2 in, 1 out]
                  n171 = call <vilib>:"Check if File or Folder Exists.vi"("path"=w236) -> ("file or folder exists?"=w237:bool, "dup path"=w238:path)  [unwired: 8 in, 1 out]
                  n172 = Equal?(x=w299, y=w305) -> (x = y?=w306:bool)
                  n173 = Equal?(x=w301, y=w302) -> (x = y?=w303:bool)
                  n174 = case shown="False" w237 {
                    tunnel: w238 -> [w322 w323]
                    tunnel: [w321 w323] -> w229
                    frame False {
                      n175 = Create Folder(path (use dialog)=w322) -> (created path=w321:path)  [unwired: 2 in, 2 out]
                    }
                    frame True {
                    }
                  }
                  n176 = Number To Decimal String(number=w308) -> (decimal integer string=w304:string)  [unwired: 1 in]
                  n177 = Number To Decimal String(number=w307) -> (decimal integer string=w300:string)  [unwired: 1 in]
                  n178 = Select(t=w305, s=w306, f=w304) -> (s? t:f=w232:string)
                  n179 = Select(t=w302, s=w303, f=w300) -> (s? t:f=w231:string)
                  n180 = Number To Decimal String(number=w278) -> (decimal integer string=w230:string)  [unwired: 1 in]
                  n181 = call "Build Text3"("T"=w230, "Index"=w233, "Length"=w232, "Width"=w231) -> ("Result"=w234:string)  [unwired: 10 in, 1 out]
                  n182 = call "Build Text"("T"=w230, "Index"=w233, "Length"=w232, "Width"=w231) -> ("Result"=w314:string)  [unwired: 10 in, 1 out]
                  n183 = local read "TRF Cluster"() -> (w271:T10)
                  n184 = local read "Compliance Cluster"() -> (w281:T6)
                  n185 = Unbundle By Name(w271) -> ("Loop Step"=w274:dbl, "First Step"=w273:dbl)
                  n186 = Build Path(base path=w229, name or relative path=w234) -> (appended path=w235:path)
                  n187 = Build Path(base path=w294, name or relative path=w314) -> (appended path=w309:path)
                  n188 = Unbundle By Name(w281) -> ("Var1 sweep settings"=w279:T15, "Var2 step settings"=w280:T16)
                  n189 = local read "TG Dielectric Prop"() -> (w223:T1)
                  n190 = Multiply(x=w274, y=w276) -> (x*y=w277:dbl)
                  n191 = local read "TRF Cluster"() -> (w286:T10)
                  n192 = local read "TRF Cluster"() -> (w289:T10)
                  n193 = call <vilib>:"Check if File or Folder Exists.vi"("path"=w235) -> ("file or folder exists?"=w212:bool, "dup path"=w213:path)  [unwired: 8 in, 1 out]
                  n194 = call <vilib>:"Check if File or Folder Exists.vi"("path"=w309) -> ("file or folder exists?"=w216:bool, "dup path"=w215:path)  [unwired: 8 in, 1 out]
                  n195 = Unbundle By Name(w223) -> ("Dielectric Constant (TG)"=w222:dbl, "Dielectric (d) (TG)"=w219:string)
                  n196 = local read "Gate Current Cluster"() -> (w228:T3)
                  n197 = Unbundle By Name(w289) -> ("Start 4"=w288:dbl, "Total Points 2"=w287:u16)
                  n198 = call "Add_File_NumExt.vi"("Extension"=".TRF" ("string"), "file or folder exists?"=w216, "Path In"=w215) -> ("Path Out"=w214:path)  [unwired: 8 in]
                  n199 = call "Add_File_NumExt.vi"("Extension"=".LKG" ("string"), "file or folder exists?"=w212, "Path In"=w213) -> ("Path Out"=w210:path)  [unwired: 8 in]
                  n200 = Unbundle By Name(w286) -> ("Start 3"=w285:dbl, "Stop 2"=w284:dbl, "Step 3"=w283:dbl)
                  n201 = Unbundle(w280) -> ("compliance (A)"=w316:dbl, "compliance (V)"=w315:dbl)
                  n202 = Add(x=w273, y=w277) -> (x+y=w272:dbl)
                  n203 = local read "TRF Cluster"() -> (w282:T10)
                  n204 = Unbundle(w279) -> ("sweep spacing (linear: 0)"=w320:u16, "sweep mode"=w319:bool, "compliance (V)"=w318:dbl, "compliance (A)"=w317:dbl)
                  n205 = local read "VISA resource name"() -> (w270:refnum<visa-resource-name>)
                  n206 = Unbundle By Name(w228) -> ("Gate Current (TRF)"=w227:T17)
                  n207 = Unbundle By Name(w282) -> ("Integration Time 3"=w267:u32)
                  n208 = Bundle By Name(cluster=w221, "Dielectric (d)"=w219) -> (w220:T9)
                  n209 = Bundle("Start 3"=w285, "Stop 2"=w284, "Step 3"=w283, "sweep spacing (linear: 0)"=w320, "sweep mode"=w319, "compliance (V)"=w318, "compliance (A)"=w317) -> (w269:T18)  [unwired: 1 in]
                  n210 = Bundle By Name(cluster=w271, "Step 4"=w272) -> (w275:T10)
                  n211 = Bundle("compliance (A)"=w316, "compliance (V)"=w315, "Start 4"=w288, "Total Points 2"=w287, w272) -> (w268:T19)  [unwired: 1 in]
                  n212 = local write "TRF Cluster"(w275) -> ()
                  n213 = local write "LKG Path"(w210) -> ()
                  n214 = local write "TRF Path"(w214) -> ()
                  n215 = call "transfer char run_subvi_SMU4_14_05_22_JWa.vi"("VISA session"=w270, "Y2 axis settings"=w227, "LKG Path"=w210, "Var1 sweep settings"=w269, "Var2 step settings"=w268, "integration time"=w267, "Input Path"=w214, "Dielectric Constant"=w222, "Sample Properties:"=w220) -> ("Check Cluster"=w264:T20, "Output"=w265:T21, "Graph Cluster"=w263:T22, "error?"=w266:errorcluster)  [unwired: 3 in]
                  n216 = local write "Vt Cluster"(w264) -> ()
                  n217 = local write "Char Cluster"(w265) -> ()
                  n218 = Unbundle By Name(w263) -> ("Linear Sqrt"=w261:cluster{dbl[], "trace":dbl[]}[], "Linear Log"=w260:cluster{dbl[], "trace":dbl[]}[], "Linear Raw"=w249:cluster{dbl[], dbl[]}[], "Saturation Sqrt"=w252:cluster{dbl[], "trace":dbl[]}[], "Saturation Log"=w251:cluster{dbl[], "trace":dbl[]}[], "Saturation Raw"=w248:cluster{dbl[], "trace":dbl[]}[], "Gate Current"=w241:cluster{dbl[], "trace":dbl[]}[])
                  n219 = local write "error out"(w266) -> ()
                  n220 = Index Array(array=w261, index=w259) -> (element=w258:cluster{dbl[], "trace":dbl[]})
                  n221 = Index Array(array=w260, index=w259) -> (element=w257:cluster{dbl[], "trace":dbl[]})
                  n222 = Index Array(array=w252, index=w253) -> (element=w254:cluster{dbl[], "trace":dbl[]})
                  n223 = Index Array(array=w251, index=w253) -> (element=w255:cluster{dbl[], "trace":dbl[]})
                  n224 = local read "Graph Cluster"() -> (w262:T7)
                  n225 = Build Array(w258, w257) -> (w256:cluster{dbl[], "trace":dbl[]}[])
                  n226 = Build Array(w254, w255) -> (w250:cluster{dbl[], "trace":dbl[]}[])
                  n227 = Bundle By Name(cluster=w262, "Linear Transfer"=w256, "Linear Raw"=w249, "Saturation Transfer"=w250, "Saturation Raw"=w248, "TRF Gate Current"=w241) -> (w247:T7)
                  n228 = local write "Graph Cluster"(w247) -> ()
                }
              }
            }
          }
        }
      }
    }
    frame #3 {
      n229 = local write "Status Indicator"(FALSE) -> ()
    }
    frame #4 {
      # "This frame creates the countdown timer for the wait inbetween the\nTransfer and Transport (if both selected)."
      n230 = disable-structure shown="Disabled" {
        frame Disabled {
          n231 = node-c288(1) -> (w344:T12)  [unwired: 1 in]
          n232 = timed-loop {
            timing: w344 -> [_]
            timing-out: [_] -> w343
            i -> [w355]
            stop <- w356 stop-if-true
            n233 = node-c288() -> ()  [unwired: 1 in, 1 out]
            n234 = local read "TRF Cluster"() -> (w349:T10)
            n235 = local read "TSP Cluster"() -> (w350:T11)
            n236 = local read "Wait Cluster"() -> (w348:T5)
            n237 = Unbundle By Name(w349) -> ("Transfer 2"=w352:bool)
            n238 = Unbundle By Name(w350) -> ("Transport"=w351:bool)
            n239 = Unbundle By Name(w348) -> ("Wait Time (s)"=w346:dbl)
            n240 = And(x=w352, y=w351) -> (x .and. y?=w360:bool)
            n241 = Select(t=w346, s=w360, f=0) -> (s? t:f=w358:dbl)
            n242 = Multiply(x=w355, y=0.001) -> (x*y=w353:dbl)
            n243 = Select(t="Waiting...", s=w360, f="Ready") -> (s? t:f=w362:string)
            n244 = Subtract(x=w358, y=w353) -> (x-y=w347:dbl)
            n245 = property on="Status Indicator" class="Bool (strict)"("BoolText.Text"=w362) -> ()  [unwired: 2 in, 2 out]
            n246 = Bundle("Wait Time (s)"=w346, w347) -> (w345:cluster{"Wait Time (s)":dbl, dbl})  [unwired: 1 in]
            n247 = Less Or Equal?(x=w347, y=0) -> (x <= y?=w356:bool)
            n248 = local write "Wait Cluster"(w345) -> ()
            n249 = node-c288() -> ()  [unwired: 1 in, 1 out]
          }
          n250 = node-c288(w343) -> ()  [unwired: 1 out]
        }
        frame Enabled {
        }
      }
      n251 = local read "Light Bathe Cluster"() -> (w331:T2)
      n252 = Unbundle By Name(w331) -> ("TRF to TSP:"=w334:bool, "TRF to TSP Duration"=w333:dbl)
      n253 = local read "VISA resource name"() -> (w332:refnum<visa-resource-name>)
      n254 = case shown="True" w334 {
        tunnel: w333 -> [_ w336]
        tunnel: w332 -> [_ w335]
        frame False {
        }
        frame True {
          n255 = flat-sequence {
            tunnel: w335 -> [w337]
            tunnel: w336 -> [w339]
            tunnel: w335 -> [w340]
            frame #0 {
              w338 = u32 1 items=["positive pulse  ", "negative pulse  ", "level high  ", "level low  "] ("trigger signal")
              n256 = call "HP415xA Op-Trigger Output.vi"("trigger signal"=w338, "VISA session"=w337) -> ()  [unwired: 2 in, 1 out]
            }
            frame #1 {
              n257 = call "Time Delay2"("Delay Time (s)"=w339) -> ()  [unwired: 10 in, 1 out]
            }
            frame #2 {
              w341 = u32 0 items=["positive pulse  ", "negative pulse  ", "level high  ", "level low  "] ("trigger signal")
              n258 = call "HP415xA Op-Trigger Output.vi"("trigger signal"=w341, "VISA session"=w340) -> ()  [unwired: 2 in, 1 out]
            }
          }
        }
      }
    }
    frame #5 {
      n259 = local read "TSP Cluster"() -> (w371:T11)
      n260 = Unbundle By Name(w371) -> ("Transport"=w370:bool)
      n261 = case shown="True" w370 {
        frame False {
        }
        frame True {
          n262 = stacked-sequence {
            frame #0 {
              w405 = "XXX"
              w409 = "XXX"
              # "TSP w/o SMU4"
              n263 = local write "Status Indicator"(TRUE) -> ()
              n264 = local read "Saved Folder:"() -> (w385:path)
              n265 = local read "Sample Properties:"() -> (w421:T9)
              n266 = property on="Status Indicator" class="Bool (strict)"("BoolText.Text"="Measuring\nTransport") -> ()  [unwired: 2 in, 2 out]
              n267 = Build Path(base path=w385, name or relative path="TSP") -> (appended path=w398:path)
              n268 = Unbundle(w421) -> ("Index (#)"=w420:string, "Index (ABC)"=w419:string, "Length"=w410:string, "Width"=w406:string, "T (K)"=w380:dbl)  [unwired: 9 out]
              n269 = Concatenate Strings(w420, w419) -> (w418:string)
              n270 = Decimal String To Number(string=w410) -> (number=w413:i32)  [unwired: 2 in, 1 out]
              n271 = Decimal String To Number(string=w406) -> (number=w412:i32)  [unwired: 2 in, 1 out]
              n272 = call <vilib>:"Check if File or Folder Exists.vi"("path"=w398) -> ("file or folder exists?"=w400:bool, "dup path"=w399:path)  [unwired: 8 in, 1 out]
              n273 = case shown="False" w400 {
                tunnel: w399 -> [w434 w435]
                tunnel: [w433 w435] -> w397
                frame False {
                  n274 = Create Folder(path (use dialog)=w434) -> (created path=w433:path)  [unwired: 2 in, 2 out]
                }
                frame True {
                }
              }
              n275 = Equal?(x=w409, y=w410) -> (x = y?=w411:bool)
              n276 = Equal?(x=w405, y=w406) -> (x = y?=w414:bool)
              n277 = Number To Decimal String(number=w413) -> (decimal integer string=w408:string)  [unwired: 1 in]
              n278 = Number To Decimal String(number=w412) -> (decimal integer string=w404:string)  [unwired: 1 in]
              n279 = Select(t=w409, s=w411, f=w408) -> (s? t:f=w407:string)
              n280 = Select(t=w405, s=w414, f=w404) -> (s? t:f=w403:string)
              n281 = call "Build Text2"("T"=w380, "Index"=w418, "Length"=w407, "Width"=w403) -> ("Result"=w402:string)  [unwired: 10 in, 1 out]
              n282 = local read "Compliance Cluster"() -> (w384:T6)
              n283 = Build Path(base path=w397, name or relative path=w402) -> (appended path=w415:path)
              n284 = Unbundle By Name(w384) -> ("Var1 sweep settings 2"=w383:T15, "Var2 step settings 2"=w382:T16)
              n285 = local read "TSP Cluster"() -> (w396:T11)
              n286 = local read "TSP Cluster"() -> (w387:T11)
              n287 = call <vilib>:"Check if File or Folder Exists.vi"("path"=w415) -> ("file or folder exists?"=w417:bool, "dup path"=w416:path)  [unwired: 8 in, 1 out]
              n288 = local read "Gate Current Cluster"() -> (w374:T3)
              n289 = Unbundle By Name(w387) -> ("Start"=w392:dbl, "Total Points"=w391:u16, "Step"=w390:dbl)
              n290 = local read "TSP Cluster"() -> (w389:T11)
              n291 = Unbundle By Name(w396) -> ("Start 2"=w395:dbl, "Stop 3"=w394:dbl, "Step 2"=w393:dbl)
              n292 = Unbundle(w382) -> ("compliance (A)"=w427:dbl, "compliance (V)"=w426:dbl)
              n293 = Unbundle(w383) -> ("sweep spacing (linear: 0)"=w432:u16, "sweep mode"=w431:bool, "compliance (V)"=w430:dbl, "compliance (A)"=w429:dbl)
              n294 = call "Add_File_NumExt.vi"("Extension"=".TSP" ("string"), "file or folder exists?"=w417, "Path In"=w416) -> ("Path Out"=w381:path)  [unwired: 8 in]
              n295 = local read "VISA resource name"() -> (w386:refnum<visa-resource-name>)
              n296 = Unbundle By Name(w374) -> ("Gate Current (TSP)"=w373:T17)
              n297 = Unbundle By Name(w389) -> ("Integration Time"=w388:u32)
              n298 = Bundle("Start 2"=w395, "Stop 3"=w394, "Step 2"=w393, "sweep spacing (linear: 0)"=w432, "sweep mode"=w431, "compliance (V)"=w430, "compliance (A)"=w429) -> (w428:T23)  [unwired: 1 in]
              n299 = Bundle("compliance (A)"=w427, "compliance (V)"=w426, "Start"=w392, "Total Points"=w391, "Step"=w390) -> (w425:T24)  [unwired: 1 in]
              n300 = local write "TSP Path"(w381) -> ()
              n301 = call "transport char run_subvi_2014_05_30_JWa.vi"("VISA session"=w386, "Y2 axis settings"=w373, "Var1 sweep settings"=w428, "Var2 step settings"=w425, "integration time"=w388, "Path"=w381, "Sample Properties:"=w421) -> ("Graph Cluster"=w379:T25, "error?"=w424:errorcluster)  [unwired: 6 in, 1 out]
              n302 = local write "error out"(w424) -> ()
              n303 = Unbundle By Name(w379) -> ("Transport"=w376:cluster{dbl[], dbl[]}[], "Gate Current"=w375:cluster{dbl[], dbl[]}[])
              n304 = local read "Graph Cluster"() -> (w378:T7)
              n305 = Bundle By Name(cluster=w378, "Transport"=w376, "TSP Gate Current"=w375) -> (w377:T7)
              n306 = local write "Graph Cluster"(w377) -> ()
            }
            frame #1 {
              n307 = local read "Gated SMU4 is..."() -> (w436:bool)
              n308 = case shown="True" w436 {
                frame False {
                }
                frame True {
                  n309 = local read "Light Bathe Cluster"() -> (w440:T2)
                  n310 = Unbundle By Name(w440) -> ("TG to BG (TSP):"=w439:bool, "TG to BG Durration 3"=w438:dbl)
                  n311 = local read "VISA resource name"() -> (w437:refnum<visa-resource-name>)
                  n312 = case shown="True" w439 {
                    tunnel: w438 -> [_ w442]
                    tunnel: w437 -> [_ w441]
                    frame False {
                    }
                    frame True {
                      n313 = flat-sequence {
                        tunnel: w441 -> [w443]
                        tunnel: w442 -> [w445]
                        tunnel: w441 -> [w446]
                        frame #0 {
                          w444 = u32 1 items=["positive pulse  ", "negative pulse  ", "level high  ", "level low  "] ("trigger signal")
                          n314 = call "HP415xA Op-Trigger Output.vi"("trigger signal"=w444, "VISA session"=w443) -> ()  [unwired: 2 in, 1 out]
                        }
                        frame #1 {
                          n315 = call "Time Delay3"("Delay Time (s)"=w445) -> ()  [unwired: 10 in, 1 out]
                        }
                        frame #2 {
                          w447 = u32 0 items=["positive pulse  ", "negative pulse  ", "level high  ", "level low  "] ("trigger signal")
                          n316 = call "HP415xA Op-Trigger Output.vi"("trigger signal"=w447, "VISA session"=w446) -> ()  [unwired: 2 in, 1 out]
                        }
                      }
                    }
                  }
                }
              }
            }
            frame #2 {
              # "TSP w/ SMU4"
              n317 = local read "Gated SMU4 is..."() -> (w448:bool)
              n318 = case shown="True" w448 {
                frame False {
                }
                frame True {
                  w484 = "XXX"
                  w488 = "XXX"
                  n319 = local write "Status Indicator"(TRUE) -> ()
                  n320 = local read "Sample Properties:"() -> (w498:T9)
                  n321 = property on="Status Indicator" class="Bool (strict)"("BoolText.Text"="     Measuring\nTransport SMU4") -> ()  [unwired: 2 in, 2 out]
                  n322 = local read "Saved Folder:"() -> (w464:path)
                  n323 = Build Path(base path=w464, name or relative path="TSP_SMU4") -> (appended path=w477:path)
                  n324 = Unbundle(w498) -> ("Index (#)"=w497:string, "Index (ABC)"=w496:string, "Length"=w489:string, "Width"=w485:string, "T (K)"=w460:dbl)  [unwired: 9 out]
                  n325 = Concatenate Strings(w497, w496) -> (w495:string)
                  n326 = Decimal String To Number(string=w489) -> (number=w492:i32)  [unwired: 2 in, 1 out]
                  n327 = Decimal String To Number(string=w485) -> (number=w491:i32)  [unwired: 2 in, 1 out]
                  n328 = call <vilib>:"Check if File or Folder Exists.vi"("path"=w477) -> ("file or folder exists?"=w479:bool, "dup path"=w478:path)  [unwired: 8 in, 1 out]
                  n329 = case shown="False" w479 {
                    tunnel: w478 -> [w511 w512]
                    tunnel: [w510 w512] -> w476
                    frame False {
                      n330 = Create Folder(path (use dialog)=w511) -> (created path=w510:path)  [unwired: 2 in, 2 out]
                    }
                    frame True {
                    }
                  }
                  n331 = Equal?(x=w488, y=w489) -> (x = y?=w490:bool)
                  n332 = Equal?(x=w484, y=w485) -> (x = y?=w493:bool)
                  n333 = Number To Decimal String(number=w492) -> (decimal integer string=w487:string)  [unwired: 1 in]
                  n334 = Number To Decimal String(number=w491) -> (decimal integer string=w483:string)  [unwired: 1 in]
                  n335 = Select(t=w488, s=w490, f=w487) -> (s? t:f=w486:string)
                  n336 = Select(t=w484, s=w493, f=w483) -> (s? t:f=w482:string)
                  n337 = call "Build Text6"("T"=w460, "Index"=w495, "Length"=w486, "Width"=w482) -> ("Result"=w481:string)  [unwired: 10 in, 1 out]
                  n338 = local read "Compliance Cluster"() -> (w463:T6)
                  n339 = Build Path(base path=w476, name or relative path=w481) -> (appended path=w494:path)
                  n340 = Unbundle By Name(w463) -> ("Var1 sweep settings 2"=w462:T15, "Var2 step settings 2"=w461:T16)
                  n341 = local read "TSP Cluster"() -> (w475:T11)
                  n342 = local read "TSP Cluster"() -> (w466:T11)
                  n343 = call <vilib>:"Check if File or Folder Exists.vi"("path"=w494) -> ("file or folder exists?"=w450:bool, "dup path"=w451:path)  [unwired: 8 in, 1 out]
                  n344 = local read "Gate Current Cluster"() -> (w454:T3)
                  n345 = Unbundle By Name(w466) -> ("Start"=w471:dbl, "Total Points"=w470:u16, "Step"=w469:dbl)
                  n346 = Unbundle By Name(w475) -> ("Start 2"=w474:dbl, "Stop 3"=w473:dbl, "Step 2"=w472:dbl)
                  n347 = local read "TSP Cluster"() -> (w468:T11)
                  n348 = Unbundle(w461) -> ("compliance (A)"=w504:dbl, "compliance (V)"=w503:dbl)
                  n349 = call "Add_File_NumExt.vi"("Extension"=".TSP" ("string"), "file or folder exists?"=w450, "Path In"=w451) -> ("Path Out"=w449:path)  [unwired: 8 in]
                  n350 = Unbundle(w462) -> ("sweep spacing (linear: 0)"=w509:u16, "sweep mode"=w508:bool, "compliance (V)"=w507:dbl, "compliance (A)"=w506:dbl)
                  n351 = local read "VISA resource name"() -> (w465:refnum<visa-resource-name>)
                  n352 = Unbundle By Name(w454) -> ("Gate Current (TSP)"=w453:T17)
                  n353 = Unbundle By Name(w468) -> ("Integration Time"=w467:u32)
                  n354 = Bundle("Start 2"=w474, "Stop 3"=w473, "Step 2"=w472, "sweep spacing (linear: 0)"=w509, "sweep mode"=w508, "compliance (V)"=w507, "compliance (A)"=w506) -> (w505:T23)  [unwired: 1 in]
                  n355 = Bundle("compliance (A)"=w504, "compliance (V)"=w503, "Start"=w471, "Total Points"=w470, "Step"=w469) -> (w502:T24)  [unwired: 1 in]
                  n356 = local write "TSP Path"(w449) -> ()
                  n357 = call "transport char run_subvi_2014_05_29_SMU4_JWa.vi"("VISA session"=w465, "Y2 axis settings"=w453, "Var1 sweep settings"=w505, "Var2 step settings"=w502, "integration time"=w467, "Path"=w449, "Sample Properties:"=w498) -> ("Graph Cluster"=w459:T25, "error?"=w501:errorcluster)  [unwired: 6 in, 1 out]
                  n358 = local write "error out"(w501) -> ()
                  n359 = Unbundle By Name(w459) -> ("Transport"=w456:cluster{dbl[], dbl[]}[], "Gate Current"=w455:cluster{dbl[], dbl[]}[])
                  n360 = local read "Graph Cluster"() -> (w458:T7)
                  n361 = Bundle By Name(cluster=w458, "Transport"=w456, "TSP Gate Current"=w455) -> (w457:T7)
                  n362 = local write "Graph Cluster"(w457) -> ()
                }
              }
            }
          }
        }
      }
    }
    frame #6 {
      n363 = local write "Status Indicator"(FALSE) -> ()
      n364 = property on="Status Indicator" class="Bool (strict)"("BoolText.Text"="Ready") -> ()  [unwired: 2 in, 2 out]
    }
    frame #7 {
      n365 = disable-structure shown="Disabled" {
        disable-tunnel: w516 -> [w518 _]
        disable-tunnel: w515 -> [w517 _]
        frame Disabled {
          n366 = node-c288(100) -> (w523:T12)  [unwired: 3 in]
          n367 = timed-loop {
            timing: w523 -> [_]
            timing-out: [_] -> w522
            tunnel: w518 -> [w534]
            tunnel: w517 -> [w533]
            tunnel: ["Stop \nCountdown"] -> _
            i -> [w539]
            stop <- w529 stop-if-true
            n368 = node-c288() -> ()  [unwired: 1 in, 1 out]
            n369 = Equal?(x=w533, y=w534) -> (x = y?=w535:bool)
            n370 = property on="Status Indicator" class="Bool (strict)"("BoolText.Text"="Waiting...") -> ()  [unwired: 2 in, 2 out]
            n371 = local read "TRF Cluster"() -> (w528:T10)
            n372 = Unbundle By Name(w528) -> ("Loop Wait"=w526:dbl)
            n373 = Select(t=0, s=w535, f=w526) -> (s? t:f=w531:dbl)
            n374 = Multiply(x=0.1, y=w539) -> (x*y=w537:dbl)
            n375 = Subtract(x=w531, y=w537) -> (x-y=w525:dbl)
            n376 = Less Or Equal To 0?(x=w525) -> (x <= 0?=w530:bool)
            n377 = Bundle("Loop Wait"=w526, w525) -> (w527:cluster{"Loop Wait":dbl, dbl})  [unwired: 1 in]
            n378 = local write "Wait Cluster"(w527) -> ()
            n379 = Or(x=w530, y="Stop \nCountdown") -> (x .or. y?=w529:bool)
            n380 = node-c288() -> ()  [unwired: 1 in, 1 out]
          }
          n381 = node-c288(w522) -> (w519:errorcluster)
          n382 = property on="Status Indicator" class="Bool (strict)"(error in=w519, "BoolText.Text"="Ready") -> ()  [unwired: 1 in, 2 out]
        }
        frame Enabled {
        }
      }
    }
  }
  n383 = local write "TRF Cluster"(w7) -> ()
  n384 = local write "VISA resource name out"(w2) -> ()
